vi "Stop Core.vi"(10 "final error code":i32, 11 "Trace Grabber Application in":refnum<class "User Interface.lvclass">) -> (3 "Trace Grabber Application out":refnum<class "User Interface.lvclass">)   [LabVIEW 2016, in "User Interface.lvlib" / "User Interface.lvclass"]
doc: "(<B>Filename</B>: Actor Framework.lvlib:Actor.lvclass:Stop Core.vi)\n\nDefines what the actor does before it stops. Use the <B>final error code</B> input to determine whether the actor shut down in response to an error.\n\nBy default, this method does nothing. A descendant class may override it to define behavior, such as shutting down any processes the actor initiated in its override of the Actor Core method."
uses:
  User Interface.lvclass
  <vilib>/ActorFramework/Actor/Actor.lvclass
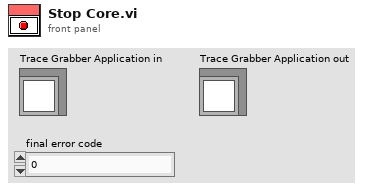
[diagram p1: front panel]
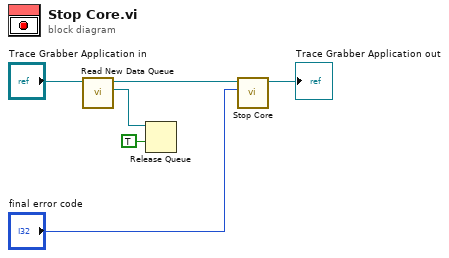
[diagram p0: block diagram]
diagram:
  n1 = call-dynamic "Read New Data Queue.vi"("User Interface in"="Trace Grabber Application in") -> ("New Data Queue"=w2:refnum<queue>, "User Interface out"=w3:refnum<class "User Interface.lvclass">)  [unwired: 9 in]
  n2 = Release Queue(queue=w2, force destroy? (F)=TRUE) -> ()  [unwired: 1 in, 3 out]
  n3 = call-parent "Stop Core.vi"("final error code"="final error code", "Actor in"=w3) -> ("Actor out"=→"Trace Grabber Application out":refnum<class "User Interface.lvclass">)  [unwired: 9 in]
